vi "findRobotClosestToPosition.vi"(8 "error in (no error)":errorcluster, 9 "robotsArray":refnum<class "Robot.lvclass">[](array[class]), 10 "position":dbl[](array[numeric]) format="%#_13g", 11 "Utilities in":refnum<class "Utilities.lvclass">) -> (0 "error out":errorcluster, 1 "Robot out":refnum<class "Robot.lvclass">, 2 "id":i32, 3 "Utilities out":refnum<class "Utilities.lvclass">, 4 "Distance":dbl)   [LabVIEW 2020, in "Utilities.lvclass"]
uses:
  Utilities.lvclass
  Robot_class/Robot.lvclass
  C:/Users/anton/Desktop/RoboIME/SSL/SSL_AI/Object_class/Object.lvclass
  Object_class/Object.lvclass/Object.ctl
  Robot_class/Robot.lvclass/Robot.ctl
  Object_class/Read position(x,y).vi
  Robot_class/Read id.vi
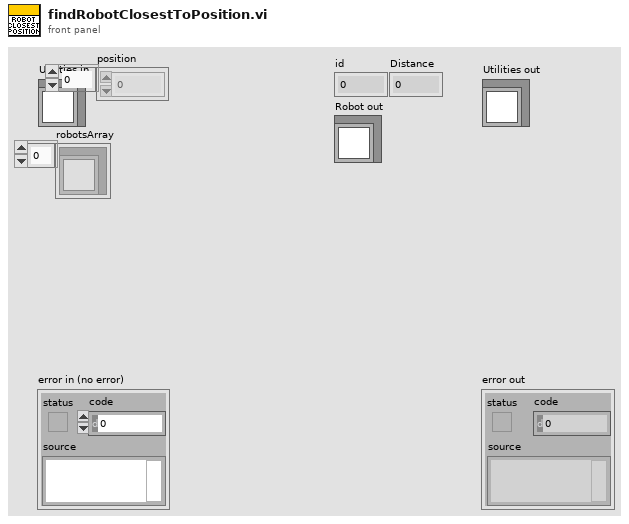
[diagram p1: front panel]
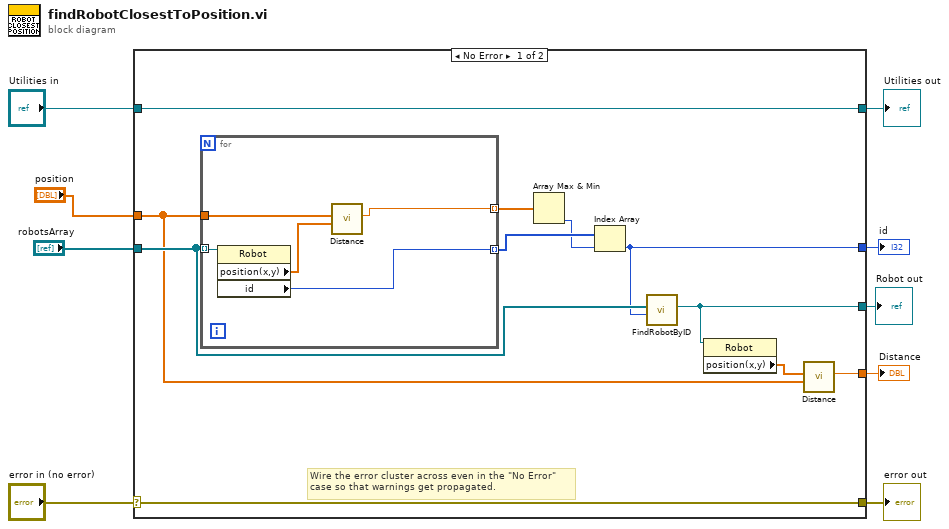
[diagram p0: block diagram]
diagram:
  n1 = case shown="No Error" "error in (no error)" {
    selector: "error in (no error)" -> [w19 w27]
    tunnel: [w19 w27] -> w8
    tunnel: [w20 w26] -> w6
    tunnel: "Utilities in" -> [w20 w26]
    tunnel: "robotsArray" -> [w15 _]
    tunnel: "position" -> [w11 _]
    tunnel: [w14 _] -> w3
    tunnel: [w13 _] -> w2
    tunnel: [w10 _] -> w1
    frame No Error {
      # "Wire the error cluster across even in the \"No Error\"\ncase so that warnings get propagated."
      n2 = for {
        tunnel: w15 -> [w24] mode=indexing
        tunnel: w11 -> [w25]
        tunnel: [w22] -> w18 mode=indexing
        tunnel: [w21] -> w17 mode=indexing
        n3 = property class="Robot"(reference=w24) -> ("position(x,y)"=w23:dbl[], "id"=w21:i32)  [unwired: 1 in, 2 out]
        n4 = call "Distance.vi"("P1"=w23, "P2"=w25) -> ("Distance"=w22:dbl)  [unwired: 7 in, 2 out]
      }
      n5 = Array Max & Min(array=w18) -> (min index (indices)=w16:i32)  [unwired: 3 out]
      n6 = Index Array(array=w17, index=w16) -> (element=w14:i32)
      n7 = call "FindRobotByID.vi"("id"=w14, "RobotRef"=w15) -> ("Robot"=w13:refnum<class "Robot.lvclass">)  [unwired: 6 in, 3 out]
      n8 = property class="Robot"(reference=w13) -> ("position(x,y)"=w12:dbl[])  [unwired: 1 in, 2 out]
      n9 = call "Distance.vi"("P1"=w11, "P2"=w12) -> ("Distance"=w10:dbl)  [unwired: 7 in, 2 out]
    }
    frame Error {
    }
  }
  "error out" <- w8
  "Utilities out" <- w6
  "id" <- w3
  "Robot out" <- w2
  "Distance" <- w1
